vi "GetSetNotifierQueue.vi"(3 "Name":enum16{"topic", "node"}(ring)=enum."node", 4 "Command":string, 5 "ROS":T1={"topic port"=0, "Node"="", "topic"="", "type"="", "node port"=0, "error "={"status"=FALSE, "code"=0, "source"=""}, "Direction"=enum."Node", "APIs"=[], "Update (ms)"=1, "write queue"=1}) -> (1 "MyState":T4, 2 "Log":T3)   [LabVIEW 2012]
uses:
  <userlib>/ROSforLV/ROS/Code/Console/Servers/ServerSubs/MyState.ctl
  <userlib>/ROSforLV/ROS/Code/Console/Servers/ServerSubs/ROSLog.ctl
  <userlib>/ROSforLV/ROS/Code/SubVIs/_ROSControl.ctl
  <userlib>/ROSforLV/ROS/Code/SubVIs/_ROSDirection.ctl
  <userlib>/ROSforLV/ROS/Code/_ROSDefinition.vi
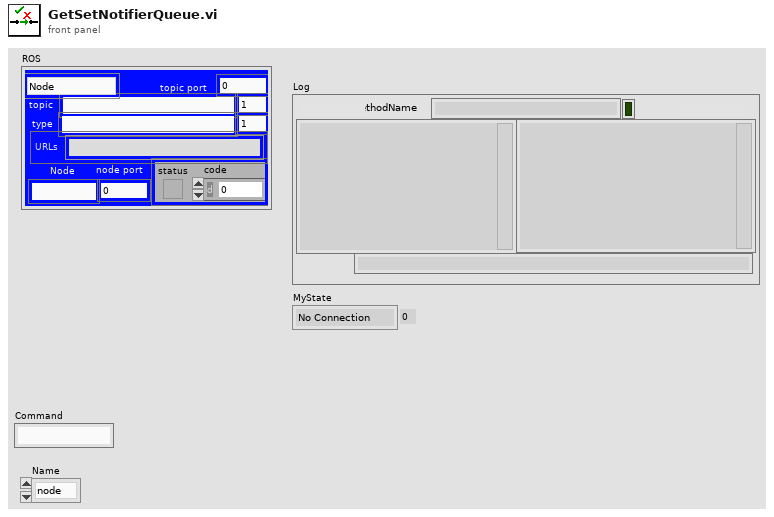
[diagram p1: front panel]
types:
  T1 = typedef "_ROSControl.ctl" = cluster{"topic port":u16, "Node":string, "topic":string, "type":string, "node port":u32, "error ":errorcluster, "Direction":T2, "APIs":string[], "Update (ms)":u16, "write queue":u16}
  T2 = typedef "_ROSDirection.ctl" = enum16{"Node", "Publisher", "Subscriber", "Service Client"}
  T3 = typedef "ROSLog.ctl" = cluster{"Sent":string, "Reply":string, "MethodName":string, "success":bool, "Dir1":string, "Dir2":string, "Time Stamp":string, "error":errorcluster, "Preamble":string}
  T4 = typedef "MyState.ctl" = enum16{"No Connection", "Registered", "Connected", "Close"}
  T5 = typedef "ServoInfo.ctl" = cluster{"vi name":string, "VI Refnum":refnum<vi>, "queue":refnum<queue>, "ROS":T1, "notifier":refnum<notifier>}
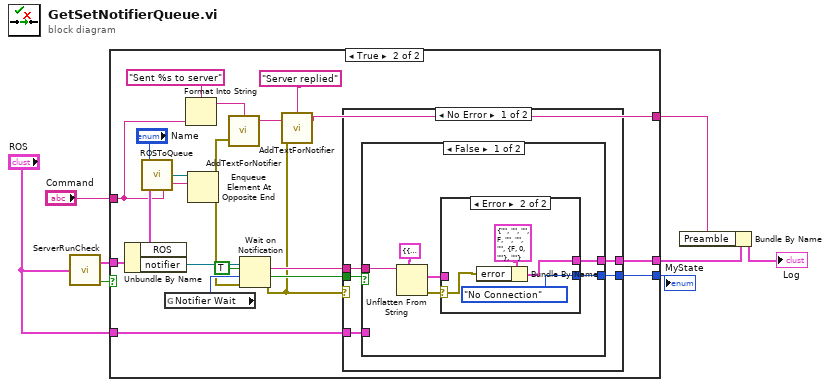
[diagram p0: block diagram]
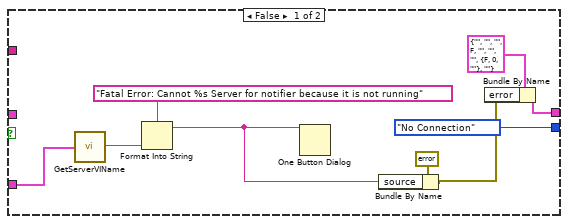
[diagram p2: hidden frame]
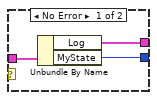
[diagram p3: hidden frame]
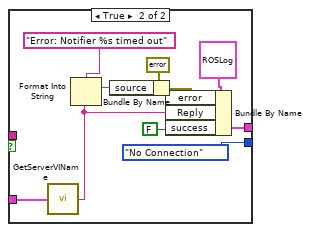
[diagram p4: hidden frame]
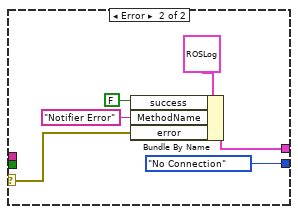
[diagram p5: hidden frame]
diagram:
  n1 = call <userlib>:"ServerRunCheck.vi"("ROS in"="ROS") -> ("Running?"=w6:bool, "ServerFound"=w5:T5)
  n2 = case shown="True" w6 {
    tunnel: w5 -> [_ w33]
    tunnel: "Command" -> [_ w25]
    tunnel: [w10 w31] -> w3
    tunnel: [MyState."No Connection" ("MyState") w30] -> w8
    tunnel: "ROS" -> [w11 w27]
    tunnel: [_ w18] -> w1
    frame False {
      n3 = call <userlib>:"GetServerVIName.vi"("ROS"=w11) -> ("vi name"=w15:string)
      n4 = Format Into String(format string="Fatal Error: Cannot %s Server for notifier because it is not running" ("message"), w15) -> (resulting string=w12:string)  [unwired: 2 in, 1 out]
      n5 = One Button Dialog(message=w12) -> ()  [unwired: 1 in, 1 out]
      n6 = Bundle By Name(cluster=errorcluster {"status"=TRUE, "code"=0, "source"=""} ("error IO"), "source"=w12) -> (w9:errorcluster)
      n7 = Bundle By Name(cluster=T3 {"Sent"="", "Reply"="", "MethodName"="", "success"=FALSE, "Dir1"="", "Dir2"="", "Time Stamp"="", "error"={"status"=FALSE, "code"=0, "source"=""}, "Preamble"=""} ("Log"), "error"=w9) -> (w10:T3)
    }
    frame True {
      n8 = Unbundle By Name(w33) -> ("ROS"=w26:T1, "notifier"=w32:refnum<notifier>)
      n9 = call <userlib>:"ROSToQueue.vi"("ROS"=w26, "Name"="Name") -> ("queue"=w29:refnum<queue>)  [unwired: 2 in, 1 out]
      n10 = global read "_ROSDefinition.vi" "Notifier Wait"() -> (w28:i32)
      n11 = Format Into String(format string="Sent %s to server", w25) -> (resulting string=w19:string)  [unwired: 2 in, 1 out]
      n12 = Enqueue Element At Opposite End(queue=w29, element=w25) -> (error out=w23:errorcluster)  [unwired: 2 in, 2 out]
      n13 = call <userlib>:"AddTextForNotifier.vi"("error in (no error)"=w23, "Command"=w19) -> ("Text out"=w20:string)  [unwired: 3 in]
      n14 = Wait on Notification(notifier=w32, ignore previous (F)=TRUE, timeout in ms (-1)=w28, error in (no error)=w23) -> (notification=w35:string, timed out?=w36:bool, error out=w22:errorcluster)  [unwired: 1 out]
      n15 = call <userlib>:"AddTextForNotifier.vi"("error in (no error)"=w22, "Text in"=w20, "Command"="Server replied" ("format string")) -> ("Text out"=w18:string)  [unwired: 2 in]
      n16 = case shown="No Error" w22 {
        selector: w22 -> [_ w69]
        tunnel: w36 -> [w42 _]
        tunnel: w35 -> [w41 _]
        tunnel: [w40 w66] -> w31
        tunnel: [w39 MyState."No Connection" ("MyState")] -> w30
        tunnel: w27 -> [w38 _]
        frame No Error {
          n17 = case shown="False" w42 {
            tunnel: w41 -> [w48 _]
            tunnel: [w46 MyState."No Connection" ("MyState")] -> w39
            tunnel: [w45 w62] -> w40
            tunnel: w38 -> [_ w64]
            frame False {
              n18 = Unflatten From String(type=cluster{"Log":T3, "MyState":T4} {"Log"={"Sent"="", "Reply"="", "MethodName"="", "success"=FALSE, "Dir1"="", "Dir2"="", "Time Stamp"="", "error"={"status"=FALSE, "code"=0, "source"=""}, "Preamble"=""}, "MyState"=enum."No Connection"} ("output cluster"), binary string=w48) -> (value=w47:cluster{"Log":T3, "MyState":T4}, error out=w44:errorcluster)  [unwired: 3 in, 1 out]
              n19 = case shown="Error" w44 {
                selector: w44 -> [_ w54]
                tunnel: w47 -> [w51 _]
                tunnel: [w50 MyState."No Connection" ("MyState")] -> w46
                tunnel: [w49 w52] -> w45
                frame No Error {
                  n20 = Unbundle By Name(w51) -> ("Log"=w49:T3, "MyState"=w50:T4)
                }
                frame Error {
                  n21 = Bundle By Name(cluster=T3 {"Sent"="", "Reply"="", "MethodName"="", "success"=FALSE, "Dir1"="", "Dir2"="", "Time Stamp"="", "error"={"status"=FALSE, "code"=0, "source"=""}, "Preamble"=""} ("Log"), "error"=w54) -> (w52:T3)
                }
              }
            }
            frame True {
              n22 = call <userlib>:"GetServerVIName.vi"("ROS"=w64) -> ("vi name"=w60:string)
              n23 = Format Into String(format string="Error: Notifier %s timed out" ("MethodName"), w60) -> (resulting string=w58:string)  [unwired: 2 in, 1 out]
              n24 = Bundle By Name(cluster=errorcluster {"status"=TRUE, "code"=0, "source"=""} ("error IO"), "source"=w58) -> (w57:errorcluster)
              n25 = Bundle By Name(cluster=T3 {"Sent"="Notifier Timed Out", "Reply"="", "MethodName"="Error", "success"=FALSE, "Dir1"="", "Dir2"="", "Time Stamp"="", "error"={"status"=FALSE, "code"=0, "source"=""}, "Preamble"=""} ("Log"), "error"=w57, "Reply"=w60, "success"=FALSE) -> (w62:T3)
            }
          }
        }
        frame Error {
          n26 = Bundle By Name(cluster=T3 {"Sent"="Notifier error", "Reply"="", "MethodName"="Error", "success"=FALSE, "Dir1"="", "Dir2"="", "Time Stamp"="", "error"={"status"=FALSE, "code"=0, "source"=""}, "Preamble"=""} ("Log"), "success"=FALSE, "MethodName"="Notifier Error", "error"=w69) -> (w66:T3)
        }
      }
    }
  }
  "MyState" <- w8
  n27 = Bundle By Name(cluster=w3, "Preamble"=w1) -> (→"Log":T3)
